vi "Unflatten UIP Value.vi"(10 "String Value":string, 11 "Template UIP In":refnum<class "PositionUIP.lvclass">) -> (0 "Error Out":errorcluster, 3 "Template UIP Out":refnum<class "PositionUIP.lvclass">)   [LabVIEW 2020, in "UIM.lvlib" / "PositionUIP.lvclass"]
uses:
  PositionUIP.lvclass
  <vilib>/Utility/miscctls.llb/LVPositionTypeDef.ctl
  PositionUIP.lvclass/PositionUIP.ctl
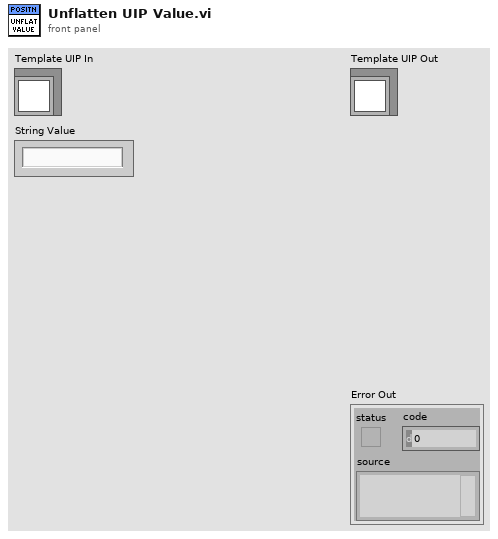
[diagram p1: front panel]
types:
  T1 = typedef "LVPositionTypeDef.ctl" = cluster{"Left":i32, "Top":i32}
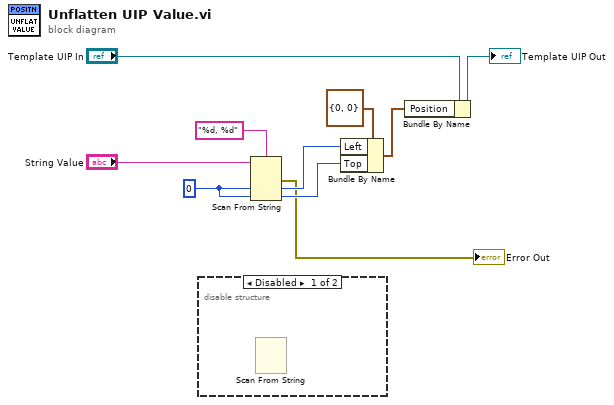
[diagram p0: block diagram]
diagram:
  w9 = 0
  n1 = disable-structure shown="Disabled" {
    frame Disabled {
      n2 = Scan From String "Scan From String"() -> ()  [unwired: 6 in, 3 out]
    }
    frame Enabled {
    }
  }
  n3 = Scan From String(format string="%d, %d", input string="String Value", default 1=w9, default 2=w9) -> (error out=→"Error Out":errorcluster, output 1=w5:i32, output 2=w4:i32)  [unwired: 2 in, 2 out]
  n4 = Bundle By Name(cluster=T1 {"Left"=0, "Top"=0} ("Position"), "Left"=w5, "Top"=w4) -> (w3:T1)
  n5 = Bundle By Name(cluster="Template UIP In", "Position"=w3) -> (→"Template UIP Out":refnum<class "PositionUIP.lvclass">)
